vi "MM_CleanUpPanel.vi"(8 "error in (no error)":errorcluster, 9 "Conpane":refnum<vi>, 11 "VI Refnum":refnum<vi>) -> (0 "error out":errorcluster)   [LabVIEW 2020]
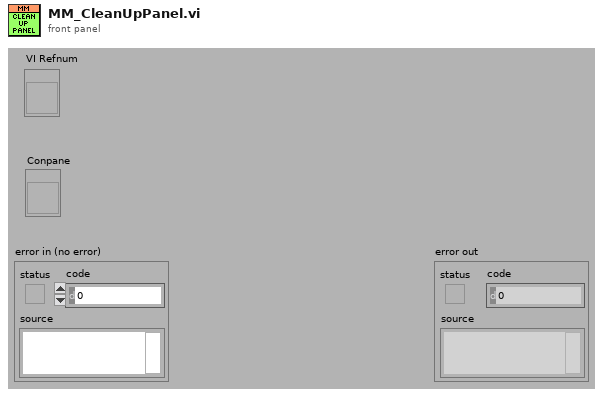
[diagram p1: front panel]
types:
  T1 = cluster{"Ctl Refnum":refnum<vi>, "width":i32, "height":i32}
  T2 = typedef "LVRectTypeDef.ctl" = cluster{"Left":i16, "Top":i16, "Right":i16, "Bottom":i16}
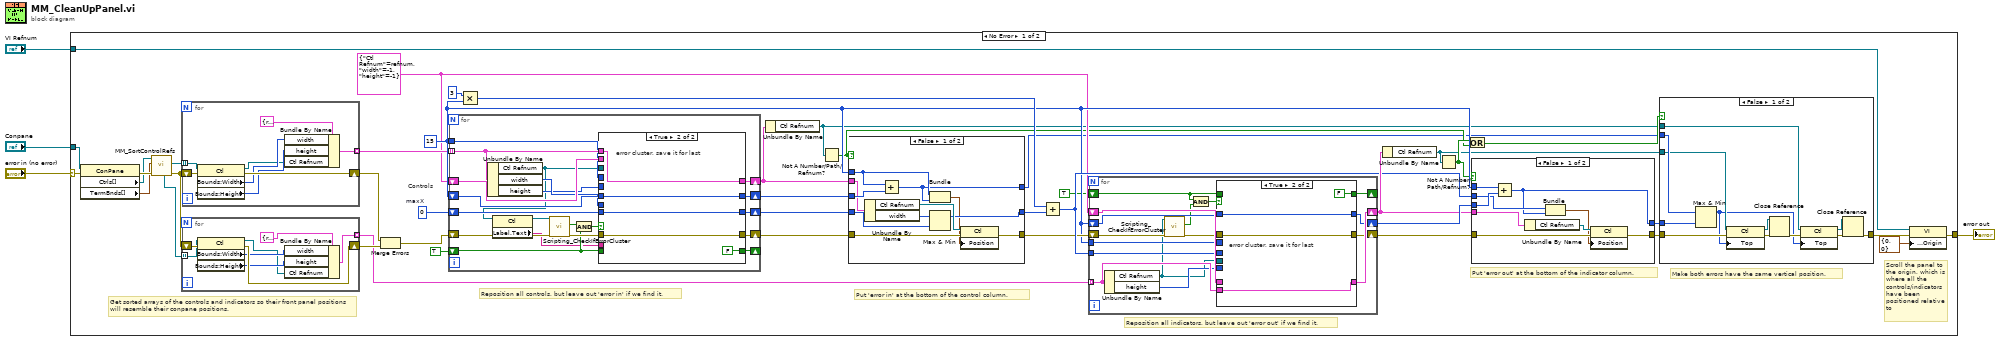
[diagram p0: block diagram]
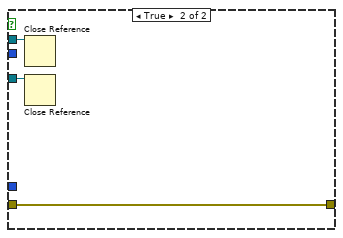
[diagram p2: hidden frame]
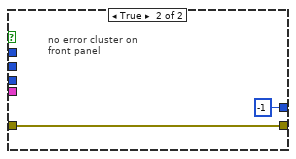
[diagram p3: hidden frame]
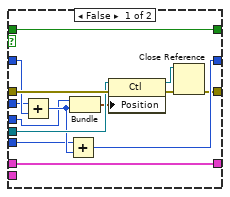
[diagram p4: hidden frame]
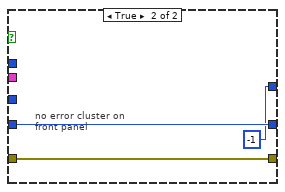
[diagram p5: hidden frame]
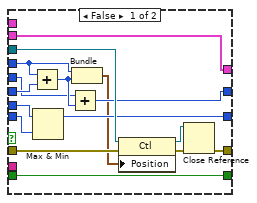
[diagram p6: hidden frame]
diagram:
  n1 = case shown="No Error" "error in (no error)" {
    selector: "error in (no error)" -> [w29 w178]
    tunnel: [w34 w178] -> w4
    tunnel: "VI Refnum" -> [w33 _]
    tunnel: "Conpane" -> [w25 _]
    frame No Error {
      w30 = 15 ("spacing")
      w16 = T1 {"Ctl Refnum"=refnum, "width"=-1, "height"=-1} ("control info prototype")
      w46 = 0  # maxX
      # "Scroll the panel to the origin, which is where all the controls/indicators have been positioned relative to"
      # "Make both errors have the same vertical position."
      # "Put 'error out' at the bottom of the indicator column."
      # "Reposition all indicators, but leave out 'error out' if we find it."
      # "Put 'error in' at the bottom of the control column."
      # "Reposition all controls, but leave out 'error in' if we find it."
      # "Get sorted arrays of the controls and indicators so their front panel positions will resemble their conpane positions."
      # "Controls"
      n2 = property class="ConPane"(reference=w25, error in=w29) -> (error out=w28:errorcluster, "Ctrls[]"=w27:refnum<vi>[], "TermBnds[]"=w26:T2[])  [unwired: 1 out]
      n3 = call "MM_SortControlRefs.vi"("error in (no error)"=w28, "Terminal Bounds[]"=w26, "Unsorted Refnums"=w27) -> ("error out"=w23:errorcluster, "Sorted Controls"=w24:refnum<vi>[], "Sorted Indicators"=w22:refnum<vi>[])  [unwired: 4 in, 2 out]
      n4 = for "Separate controls and indicators" {
        shift-right: [w176] -> w21
        shift-left: w23 -> [w177]
        tunnel: [w171] -> w18 mode=indexing
        tunnel: w24 -> [w170] mode=indexing
        n5 = property class="Ctl"(reference=w170, error in=w177) -> (reference out=w173:refnum<vi>, error out=w176:errorcluster, "Bounds:Width"=w175:u32, "Bounds:Height"=w174:u32)
        n6 = Bundle By Name(cluster=T1 {"Ctl Refnum"=refnum, "width"=0, "height"=0} ("control info prototype"), "width"=w175, "height"=w174, "Ctl Refnum"=w173) -> (w171:T1)
      }
      n7 = for "Separate controls and indicators" {
        shift-right: [w68] -> w20
        shift-left: w23 -> [w69]
        tunnel: [w63] -> w17 mode=indexing
        tunnel: w22 -> [w62] mode=indexing
        n8 = property class="Ctl"(reference=w62, error in=w69) -> (reference out=w65:refnum<vi>, error out=w68:errorcluster, "Bounds:Width"=w67:u32, "Bounds:Height"=w66:u32)
        n9 = Bundle By Name(cluster=T1 {"Ctl Refnum"=refnum, "width"=0, "height"=0} ("control info prototype"), "width"=w67, "height"=w66, "Ctl Refnum"=w65) -> (w63:T1)
      }
      n10 = Merge Errors(w21, w20) -> (w19:errorcluster)
      n11 = for "position controls" {
        shift-right: [w143] -> w44
        shift-left: w19 -> [w137]
        shift-right: [w145] -> w35
        shift-left: w16 -> [w146]
        tunnel: w18 -> [w144] mode=indexing
        shift-right: [w147] -> w43
        shift-left: w46 -> [w148]
        shift-right: [w141] -> w42
        shift-left: w30 -> [w142]
        tunnel: w30 -> [w138]
        shift-right: [w135] -> _
        shift-left: TRUE -> [w133]
        n12 = Unbundle By Name(w144) -> ("Ctl Refnum"=w131:refnum<vi>, "width"=w140:i32, "height"=w139:i32)
        n13 = property class="Ctl"(reference=w131) -> (reference out=w129:refnum<vi>, "Label.Text"=w130:string)  [unwired: 1 in, 1 out]
        n14 = call "Scripting_CheckIfErrorCluster.vi"("error in (no error)"=w137, "Ctl Refnum"=w129) -> ("error out"=w136:errorcluster, "IsErrClust?"=w134:bool)  [unwired: 7 in, 1 out]
        n15 = And(x=w134, y=w133) -> (x .and. y?=w132:bool)
        n16 = case shown="True" w132 {
          tunnel: w148 -> [w161 w169]
          tunnel: [w159 w169] -> w147
          tunnel: w146 -> [w164 _]
          tunnel: [w164 w168] -> w145
          tunnel: w144 -> [_ w168]
          tunnel: w136 -> [w163 w167]
          tunnel: [w153 w167] -> w143
          tunnel: w142 -> [w158 w166]
          tunnel: [w154 w166] -> w141
          tunnel: w140 -> [w160 _]
          tunnel: w139 -> [w155 _]
          tunnel: w131 -> [w162 _]
          tunnel: w138 -> [w157 _]
          tunnel: [w149 FALSE] -> w135
          tunnel: w133 -> [w149 _]
          tunnel: w130 -> [_ _]
          frame False {
            n17 = Add(x=w157, y=w158) -> (x+y=w156:i32)
            n18 = Max & Min(x=w160, y=w161) -> (max(x,y)=w159:i32)  [unwired: 1 out]
            n19 = Add(x=w155, y=w156) -> (x+y=w154:i32)
            n20 = Bundle("spacing"=w157, w156) -> (w150:cluster{"spacing":i32, i32})  [unwired: 1 in]
            n21 = property class="Ctl"(reference=w162, error in=w163, "Position"=w150) -> (reference out=w151:refnum<vi>, error out=w152:errorcluster)
            n22 = Close Reference(reference=w151, error in (no error)=w152) -> (error out=w153:errorcluster)
          }
          frame True {
            # "error cluster, save it for last"
          }
        }
      }
      n23 = Multiply(x=3, y=w30) -> (x*y=w37:i32)
      n24 = Unbundle By Name(w35) -> ("Ctl Refnum"=w7:refnum<vi>)
      n25 = Not A Number/Path/Refnum?(number/path/refnum=w7) -> (NaN/Path/Refnum?=w14:bool)
      n26 = case "place error cluster last" shown="False" w14 {
        tunnel: w35 -> [w122 _]
        tunnel: w44 -> [w123 w127]
        tunnel: w43 -> [w124 w128]
        tunnel: w42 -> [w125 _]
        tunnel: [w118 w128] -> w41
        tunnel: [w115 w127] -> w31
        tunnel: w30 -> [w119 _]
        tunnel: [w116 -1] -> w10
        frame False {
          n27 = Unbundle By Name(w122) -> ("Ctl Refnum"=w121:refnum<vi>, "width"=w120:i32)
          n28 = Add(x=w119, y=w125) -> (x+y=w116:i32)
          n29 = Bundle("spacing"=w119, w116) -> (w117:cluster{"spacing":i32, i32})  [unwired: 1 in]
          n30 = Max & Min(x=w120, y=w124) -> (max(x,y)=w118:i32)  [unwired: 1 out]
          n31 = property class="Ctl"(reference=w121, error in=w123, "Position"=w117) -> (error out=w115:errorcluster)  [unwired: 1 out]
        }
        frame True {
          # "no error cluster on\nfront panel"
        }
      }
      n32 = Add(x=w37, y=w41) -> (x+y=w36:i32)
      n33 = for "position indicators" {
        shift-right: [w93] -> w39
        shift-left: w31 -> [w87]
        shift-right: [w95] -> w38
        shift-left: w16 -> [w96]
        tunnel: w17 -> [w94] mode=indexing
        shift-right: [w88] -> w40
        shift-left: w30 -> [w92]
        tunnel: w30 -> [w90]
        tunnel: w36 -> [w89]
        shift-right: [w84] -> _
        shift-left: TRUE -> [w82]
        n34 = Unbundle By Name(w94) -> ("Ctl Refnum"=w85:refnum<vi>, "height"=w91:i32)
        n35 = call "Scripting_CheckIfErrorCluster.vi"("error in (no error)"=w87, "Ctl Refnum"=w85) -> ("error out"=w86:errorcluster, "IsErrClust?"=w83:bool)  [unwired: 7 in, 1 out]
        n36 = And(x=w82, y=w83) -> (x .and. y?=w81:bool)
        n37 = case shown="True" w81 {
          tunnel: w89 -> [w102 _]
          tunnel: w96 -> [w110 _]
          tunnel: [w110 w114] -> w95
          tunnel: w94 -> [_ w114]
          tunnel: w86 -> [w109 w113]
          tunnel: [w99 w113] -> w93
          tunnel: w92 -> [w107 w112]
          tunnel: [w103 w112] -> w88
          tunnel: w91 -> [w104 _]
          tunnel: w85 -> [w108 _]
          tunnel: w90 -> [w106 _]
          tunnel: w82 -> [w97 _]
          tunnel: [w97 FALSE] -> w84
          frame False {
            n38 = Add(x=w106, y=w107) -> (x+y=w105:i32)
            n39 = Add(x=w104, y=w105) -> (x+y=w103:i32)
            n40 = Bundle(w102, w105) -> (w98:cluster{i32, i32})  [unwired: 1 in]
            n41 = property class="Ctl"(reference=w108, error in=w109, "Position"=w98) -> (reference out=w100:refnum<vi>, error out=w101:errorcluster)
            n42 = Close Reference(reference=w100, error in (no error)=w101) -> (error out=w99:errorcluster)
          }
          frame True {
            # "error cluster, save it for last"
          }
        }
      }
      n43 = Unbundle By Name(w38) -> ("Ctl Refnum"=w8:refnum<vi>)
      n44 = Not A Number/Path/Refnum?(number/path/refnum=w8) -> (NaN/Path/Refnum?=w15:bool)
      n45 = Or(x=w15, y=w14) -> (x .or. y?=w13:bool)
      n46 = case "place error cluster last" shown="False" w15 {
        tunnel: w38 -> [w76 _]
        tunnel: w39 -> [w77 w80]
        tunnel: w40 -> [w78 _]
        tunnel: [w70 w80] -> w12
        tunnel: w30 -> [w74 _]
        tunnel: w36 -> [w73 _]
        tunnel: [w71 -1] -> w11
        frame False {
          n47 = Add(x=w74, y=w78) -> (x+y=w71:i32)
          n48 = Unbundle By Name(w76) -> ("Ctl Refnum"=w75:refnum<vi>)
          n49 = Bundle(w73, w71) -> (w72:cluster{i32, i32})  [unwired: 1 in]
          n50 = property class="Ctl"(reference=w75, error in=w77, "Position"=w72) -> (error out=w70:errorcluster)  [unwired: 1 out]
        }
        frame True {
          # "no error cluster on\nfront panel"
        }
      }
      n51 = case shown="False" w13 {
        tunnel: w12 -> [w56 w61]
        tunnel: w11 -> [w57 _]
        tunnel: w10 -> [w58 _]
        tunnel: [w50 w61] -> w9
        tunnel: w8 -> [w55 w60]
        tunnel: w7 -> [w47 w59]
        frame False {
          n52 = Max & Min(x=w58, y=w57) -> (max(x,y)=w48:i32)  [unwired: 1 out]
          n53 = property class="Ctl"(reference=w55, error in=w56, "Top"=w48) -> (reference out=w53:refnum<vi>, error out=w54:errorcluster)
          n54 = Close Reference(reference=w53, error in (no error)=w54) -> (error out=w49:errorcluster)
          n55 = property class="Ctl"(reference=w47, error in=w49, "Top"=w48) -> (reference out=w52:refnum<vi>, error out=w51:errorcluster)
          n56 = Close Reference(reference=w52, error in (no error)=w51) -> (error out=w50:errorcluster)
        }
        frame True {
          n57 = Close Reference(reference=w59) -> ()  [unwired: 1 in, 1 out]
          n58 = Close Reference(reference=w60) -> ()  [unwired: 1 in, 1 out]
        }
      }
      n59 = property class="VI"(reference=w33, error in=w9, "Front Panel Window:Origin"=cluster{"Horizontal":i16, "Vertical":i16} {"Horizontal"=0, "Vertical"=0}) -> (error out=w34:errorcluster)  [unwired: 1 out]
    }
    frame Error {
    }
  }
  "error out" <- w4
